vi "osa_save data to disk.vi"(8 "error in (no error)":errorcluster, 10 "data":u32[](array[numeric]), 11 "data file refnum in":refnum<file>) -> (0 "error out":errorcluster, 3 "data file refnum out":refnum<file>)   [LabVIEW 2021]
panel:
  # "OSA subVI: save single row of data to disk"
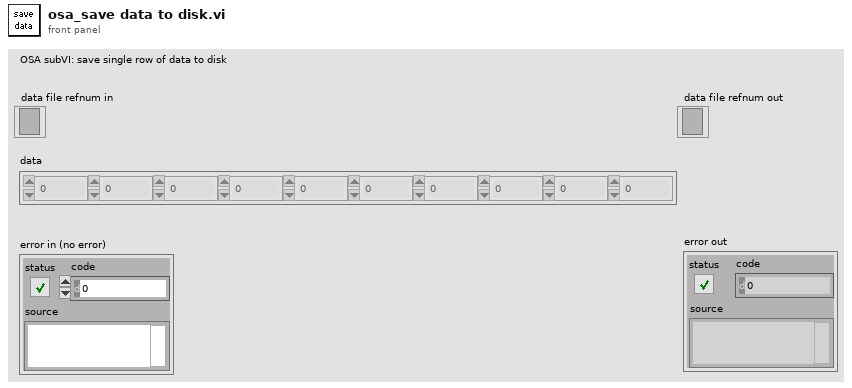
[diagram p1: front panel]
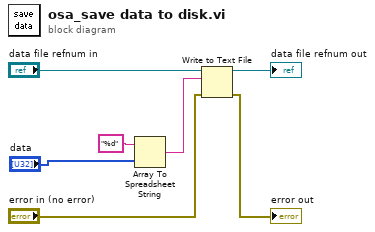
[diagram p0: block diagram]
diagram:
  n1 = Array To Spreadsheet String(array="data", 3:"%d") -> (spreadsheet string=w6:string)  [unwired: 1 in]
  n2 = Write to Text File(file (use dialog)="data file refnum in", text=w6, error in="error in (no error)") -> (refnum out=→"data file refnum out":refnum<file>, error out=→"error out":errorcluster)  [unwired: 1 in, 1 out]
